vi "Configure DST.vi"(0 "VISA resource name":refnum<visa-resource-name>, 5 "Enable DST (Disable)":bool, 7 "Start Time":T2={"Month (Mar)"=3, "Week (2nd)"=2, "Weekday (Sun)"=0, "Hour (2)"=2} {"Hour (2)" min=0 max=23; "Weekday (Sun)" items=["Sun", "Mon", "Tue", "Wed", "Thu", "Fri", "Sat"]; "Week (2nd)" items=["1st"=1, "2nd"=2, "3rd"=3, "4th"=4, "Last"=5]; "Month (Mar)" items=["Jan"=1, "Feb"=2, "Mar"=3, "Apr"=4, "May"=5, "Jun"=6, "Jul"=7, "Aug"=8, "Sep"=9, "Oct"=10, "Nov"=11, "Dec"=12]}, 9 "End Time":T1={"Month (Nov)"=11, "Week (1st)"=1, "Weekday (Sun)"=0, "Hour (2)"=2} {"Hour (2)" min=0 max=23; "Weekday (Sun)" items=["Sun", "Mon", "Tue", "Wed", "Thu", "Fri", "Sat"]; "Week (1st)" items=["1st"=1, "2nd"=2, "3rd"=3, "4th"=4, "Last"=5]; "Month (Nov)" items=["Jan"=1, "Feb"=2, "Mar"=3, "Apr"=4, "May"=5, "Jun"=6, "Jul"=7, "Aug"=8, "Sep"=9, "Oct"=10, "Nov"=11, "Dec"=12]}, 11 "error in (no error)":errorcluster) -> (4 "VISA resource name out":refnum<visa-resource-name>, 15 "error out":errorcluster)   [LabVIEW 2020, in "Yokogawa GX Series.lvlib"]
doc: "Sets the daylight saving time.\n\nCommand: SDst"
uses:
  <instrlib>/Yokogawa GX Series/Yokogawa GX Series.lvlib
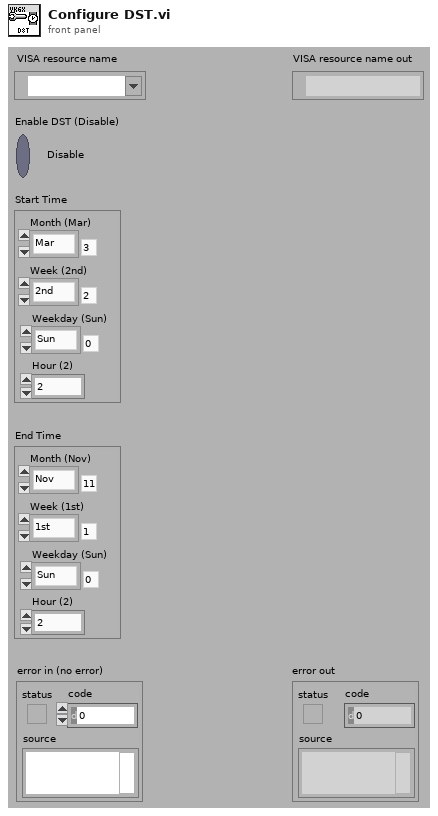
[diagram p1: front panel]
types:
  T1 = cluster{"Month (Nov)":u16, "Week (1st)":u16, "Weekday (Sun)":u16, "Hour (2)":i32}
  T2 = cluster{"Month (Mar)":u16, "Week (2nd)":u16, "Weekday (Sun)":u16, "Hour (2)":i32}
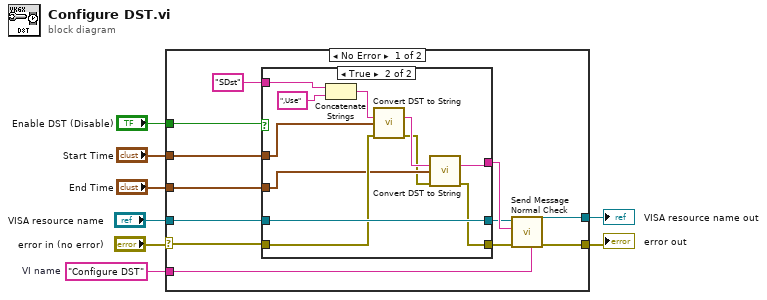
[diagram p0: block diagram]
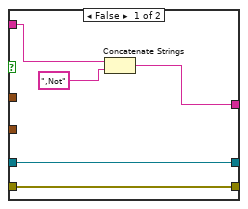
[diagram p2: hidden frame]
diagram:
  w8 = "Configure DST"  # VI name
  n1 = case shown="No Error" "error in (no error)" {
    selector: "error in (no error)" -> [w9 w37]
    tunnel: w8 -> [w20 _]
    tunnel: [w19 w38] -> w7
    tunnel: [w18 w37] -> w6
    tunnel: "Enable DST (Disable)" -> [w17 _]
    tunnel: "Start Time" -> [w14 _]
    tunnel: "End Time" -> [w13 _]
    tunnel: "VISA resource name" -> [w12 w38]
    frame No Error {
      n2 = case shown="True" w17 {
        tunnel: "SDst" -> [w25 w35]
        tunnel: [w23 w26] -> w15
        tunnel: w14 -> [_ w33]
        tunnel: w13 -> [_ w29]
        tunnel: w12 -> [w22 w32]
        tunnel: [w22 w32] -> w11
        tunnel: w9 -> [w21 w31]
        tunnel: [w21 w27] -> w10
        frame False {
          n3 = Concatenate Strings(w25, ",Not") -> (w23:string)
        }
        frame True {
          n4 = Concatenate Strings(w35, ",Use") -> (w34:string)
          n5 = call <instrlib>:"Convert DST to String.vi"("Initial string"=w34, "Time"=w33, "error in (no error)"=w31) -> ("Resulting string"=w30:string, "error out"=w28:errorcluster)  [unwired: 11 in]
          n6 = call <instrlib>:"Convert DST to String.vi"("Initial string"=w30, "Time"=w29, "error in (no error)"=w28) -> ("Resulting string"=w26:string, "error out"=w27:errorcluster)  [unwired: 11 in]
        }
      }
      n7 = call <instrlib>:"Send Message Normal Check.vi"("Source (\"\")"=w20, "error in (no error)"=w10, "Send Message (\"\")"=w15, "VISA resource name"=w11) -> ("error out"=w18:errorcluster, "VISA resource name out"=w19:refnum<visa-resource-name>)  [unwired: 2 in, 4 out]
    }
    frame Error {
    }
  }
  "error out" <- w6
  "VISA resource name out" <- w7
